vi "Read TEDS Status.vi"(11 "ILC in":refnum<class "ILC.lvclass">) -> (2 "TEDS Status":string, 3 "ILC out":refnum<class "ILC.lvclass">)   [LabVIEW 2015, in "ILCCommon.lvlib" / "ILC.lvclass"]
uses:
  <userlib>/Common/ILC/ILC/ILC.lvclass
  <userlib>/Common/ILC/ILC/ILC.lvclass/ILC.ctl
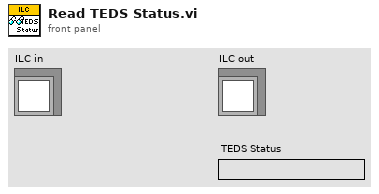
[diagram p1: front panel]
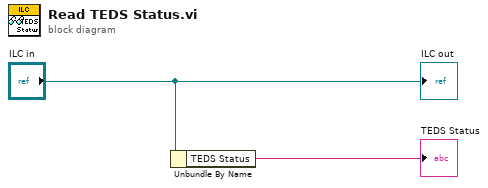
[diagram p0: block diagram]
diagram:
  n1 = Unbundle By Name("ILC in") -> ("TEDS Status"=→"TEDS Status":string)
  "ILC out" <- "ILC in"
